vi "P7.vi"() -> ()   [LabVIEW 2018]
panel:
  out "2D Picture":picture
  out "error out":errorcluster
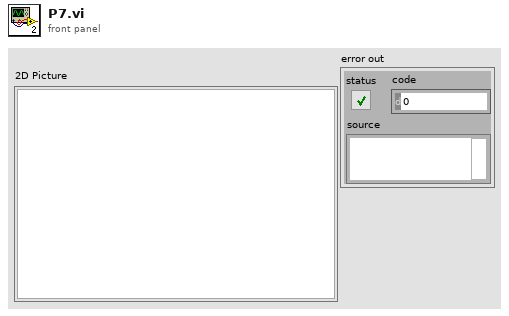
[diagram p1: front panel]
types:
  T1 = typedef "imagedata.ctl" = cluster{"image type":i32, "image depth":i32, "image":u8[], "mask":u8[], "colors":u32[], "Rectangle":cluster{"left":i16, "top":i16, "right":i16, "bottom":i16}}
  T2 = cluster{"image type":u32, "image depth":u32, "image":u32[], "mask":u32[], "colors":u32[], "Rectangle":cluster{"left":u32, "top":u32, "right":u32, "bottom":u32}}
  T3 = typedef "LVBoundsTypeDef.ctl" = cluster{"Width":u32, "Height":u32}
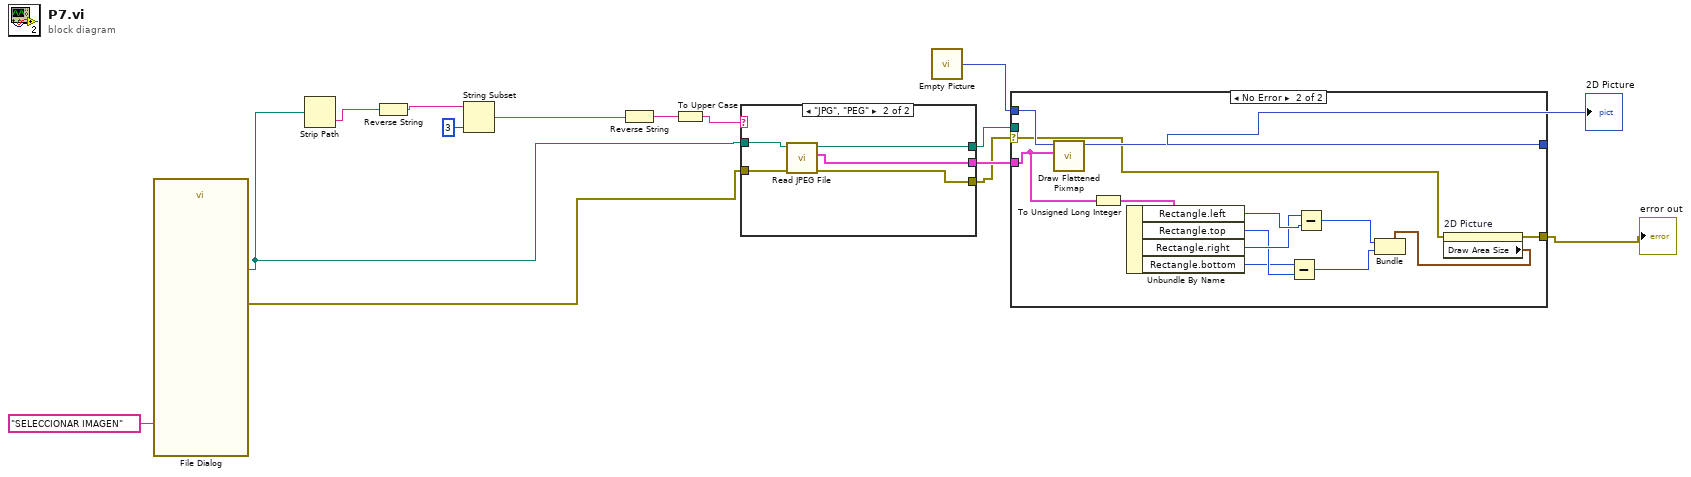
[diagram p0: block diagram]
diagram:
  n1 = call "File Dialog"("prompt"="SELECCIONAR IMAGEN") -> ("selected path"=w8:path, "error out"=w9:errorcluster)  [unwired: 11 in, 2 out]
  n2 = Strip Path(path=w8) -> (name=w14:string)  [unwired: 1 out]
  n3 = Reverse String(1:w14) -> (0:w13:string)
  n4 = String Subset(string=w13, length (rest)=3 ("length (rest)")) -> (substring=w11:string)  [unwired: 1 in]
  n5 = Reverse String(1:w11) -> (0:w10:string)
  n6 = To Upper Case(1:w10) -> (0:w3:string)
  n7 = case shown="\"JPG\", \"PEG\"" w3 {
    tunnel: [_ w21] -> w6
    tunnel: [_ w20] -> w7
    tunnel: [w16 w19] -> w2
    tunnel: w9 -> [w16 w18]
    tunnel: w8 -> [_ w17]
    frame "False", Default {
    }
    frame "JPG", "PEG" {
      n8 = call <vilib>:"Read JPEG File.vi"("error in (no error)"=w18, "path to JPEG file"=w17) -> ("error out"=w19:errorcluster, "image data"=w20:T1, "path"=w21:path)  [unwired: 7 in]
    }
  }
  n9 = call "Empty Picture"() -> ("empty picture"=w5:picture)
  n10 = case shown="No Error" w2 {
    selector: w2 -> [w23 w26]
    tunnel: w7 -> [_ w34]
    tunnel: w6 -> [_ _]
    tunnel: w5 -> [w22 w35]
    tunnel: [w22 w36] -> w4
    tunnel: [_ w25] -> w1
    frame Error {
    }
    frame No Error {
      n11 = call <vilib>:"Draw Flattened Pixmap.vi"("image data"=w34, "picture"=w35) -> ("new picture"=w36:picture)  [unwired: 7 in]
      n12 = To Unsigned Long Integer(number=w34) -> (unsigned 32bit integer=w33:T2)
      n13 = Unbundle By Name(w33) -> ("Rectangle.left"=w30:u32, "Rectangle.top"=w28:u32, "Rectangle.right"=w29:u32, "Rectangle.bottom"=w27:u32)
      n14 = Subtract(x=w27, y=w28) -> (x-y=w31:u32)
      n15 = Subtract(x=w29, y=w30) -> (x-y=w32:u32)
      n16 = property on="2D Picture" class="Pict"(error in=w26) -> (error out=w25:errorcluster, "Draw Area Size"=w24:T3)  [unwired: 1 in, 1 out]
      n17 = Bundle(cluster=w24, "Width"=w32, "Height"=w31) -> ()  [unwired: 1 out]
    }
  }
  "error out" <- w1
  "2D Picture" <- w4
